vi "XML - Get XML file name.vi"(8 "error in (no error)":errorcluster, 10 "CD Execution Mode (Asynchronous)":T1, 11 "CD Name":string="NewCD") -> (0 "error out":errorcluster, 3 "XML file name":string="Timing and Sync NewCD.xml")   [LabVIEW 2015]
doc: "Determines the file name of the XML file based on the name and execution mode of the custom device."
uses:
  TypDef/CD Wizard - Execution Mode.ctl
  Constants/Constants TypDef/XML File.ctl
  <vilib>/NI Veristand/Custom Device API/Custom Device Execution Mode.ctl
  Constants/XML File.vi
  <vilib>/NI Veristand/Custom Device API/Custom Device API.lvlib
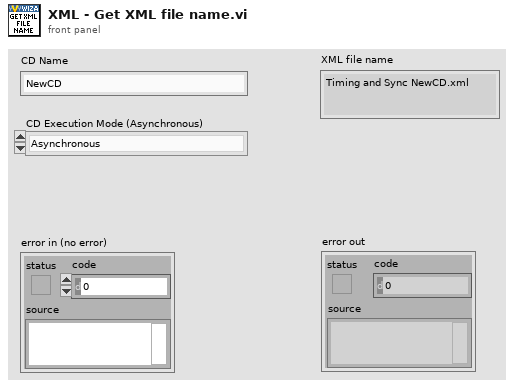
[diagram p1: front panel]
types:
  T1 = typedef "CD Wizard - Execution Mode.ctl" = enum16{"Asynchronous", "Inline HW Interface", "Inline Model Interface", "Inline Timing and Sync", "Asynchronous Timing and Sync"}
  T2 = typedef "Custom Device API.lvlib/Custom Device Execution Mode.ctl" = enum16{"Asynchronous", "Inline HW Interface", "Inline Model Interface", "Inline Timing and Sync", "Asynchronous Timing and Sync"}
  T3 = typedef "XML File.ctl" = enum16{"XMLTemplateFilePathAndName", "XMLTimingAndSyncFileName", "XMLCustomDeviceFileName"}
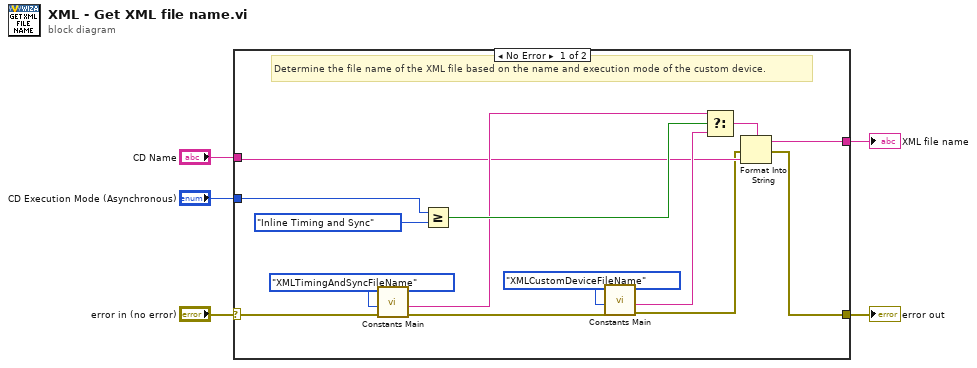
[diagram p0: block diagram]
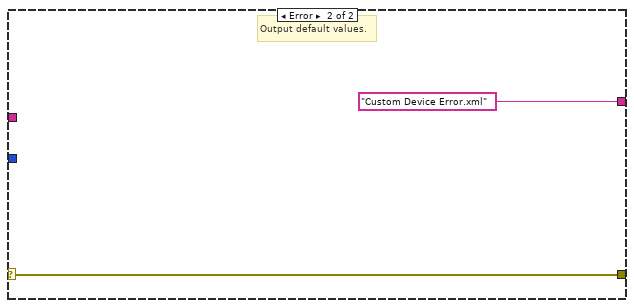
[diagram p2: hidden frame]
diagram:
  n1 = case shown="No Error" "error in (no error)" {
    selector: "error in (no error)" -> [w11 w21]
    tunnel: "CD Name" -> [w10 _]
    tunnel: "CD Execution Mode (Asynchronous)" -> [w9 _]
    tunnel: [w7 w21] -> w2
    tunnel: [w6 "Custom Device Error.xml"] -> w1
    frame No Error {
      # "Determine the file name of the XML file based on the name and execution mode of the custom device."
      n2 = call-poly "Constants Main.vi"("error in (no error)"=w11, "Action"=XML_File."XMLTimingAndSyncFileName") -> ("error out"=w14:errorcluster, "Output"=w13:string)  [unwired: 8 in]
      n3 = Greater Or Equal?(x=w9, y=Custom_Device_Execution_Mode."Inline Timing and Sync") -> (x >= y?=w15:bool)
      n4 = call-poly "Constants Main.vi"("error in (no error)"=w14, "Action"=XML_File."XMLCustomDeviceFileName") -> ("error out"=w8:errorcluster, "Output"=w12:string)  [unwired: 8 in]
      n5 = Select(t=w13, s=w15, f=w12) -> (s? t:f=w19:string)
      n6 = Format Into String(format string=w19, error in=w8, w10) -> (resulting string=w6:string, error out=w7:errorcluster)  [unwired: 1 in]
    }
    frame Error {
      # "Output default values."
    }
  }
  "error out" <- w2
  "XML file name" <- w1
